vi "Process.vi"(0 "reference in":refnum<class "Graph.lvclass">, 5 "error in":errorcluster) -> (14 "reference out":refnum<class "Graph.lvclass">, 19 "error out":errorcluster)   [LabVIEW 2023, in "Graph.lvclass"]
uses:
  Graph.lvclass
  <vilib>/Utility/SystemLogging/NI_SystemLogging.lvlib
panel:
  out "error info":errorcluster
  out "Last Command":string
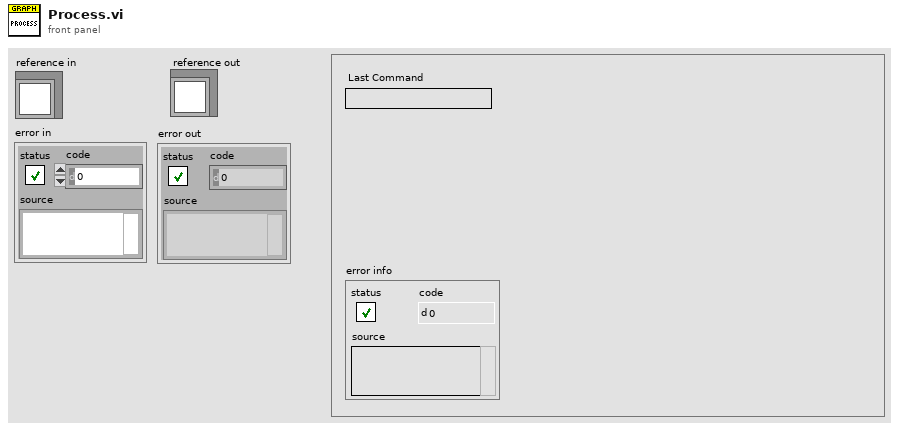
[diagram p1: front panel]
types:
  T1 = cluster{"Core":cluster{"Timeout":i32, "Events":cluster{"EventsToProcess":refnum<event-registration>}, "EventFromProcess":refnum<user-event>, "ProcessSyncQueue":refnum<queue>, "QueueFromProcess":refnum<queue>, "Command":string, "Data":variant}}
  T2 = enum32{"Invalid", "Standard", "Closed", "Hidden", "Minimized", "Maximized"}
  T3 = cluster{"EventsToProcess":refnum<event-registration>}
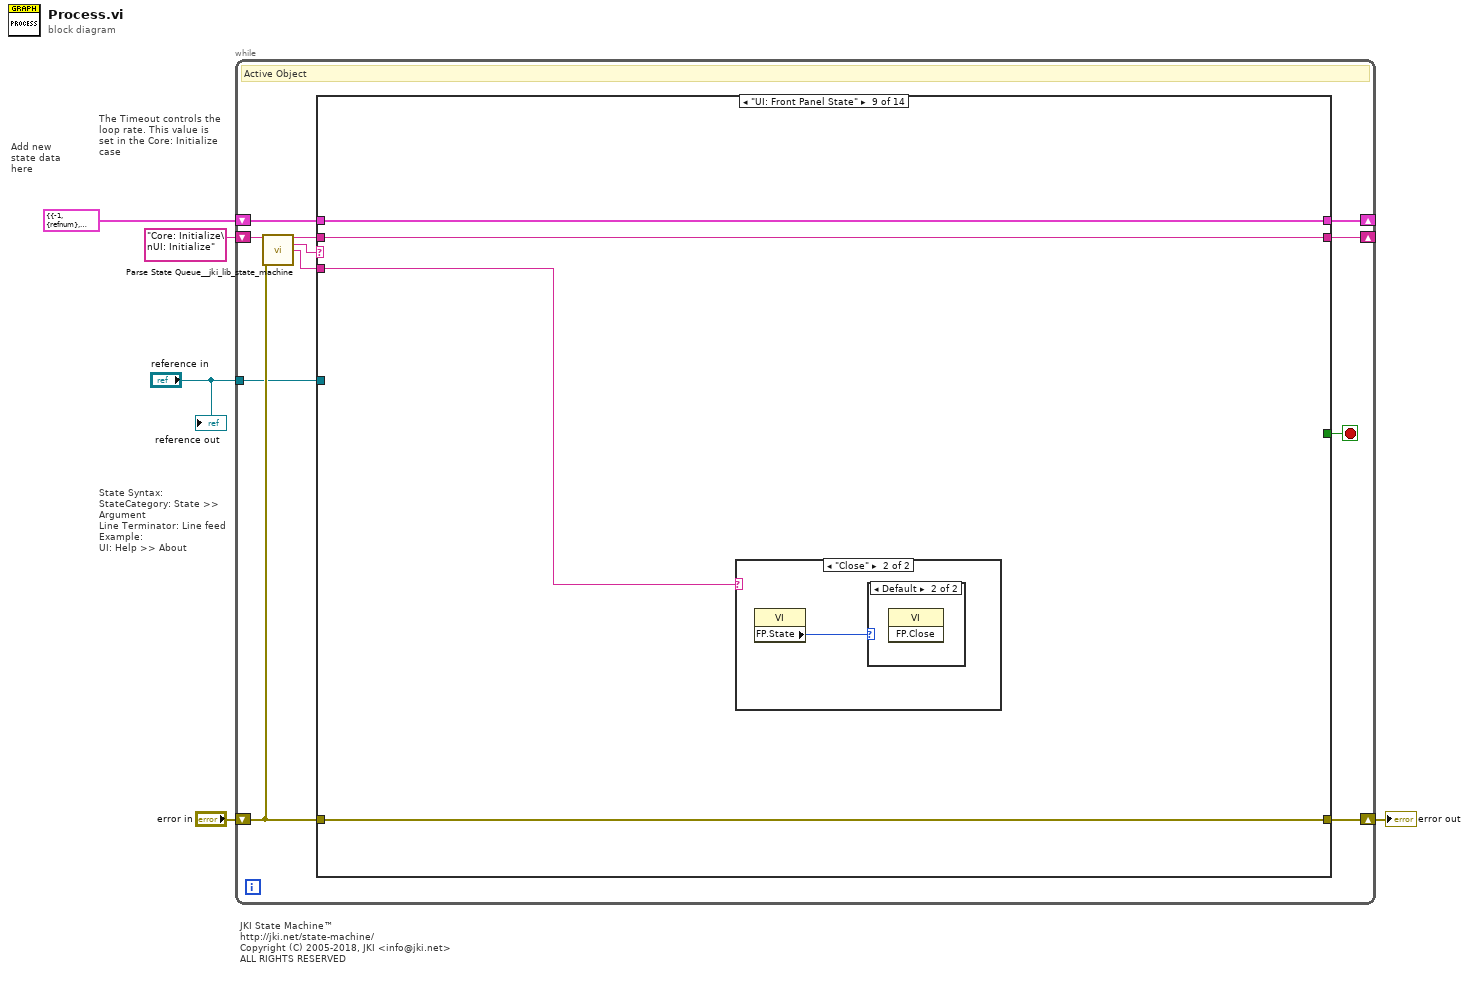
[diagram p0: block diagram]
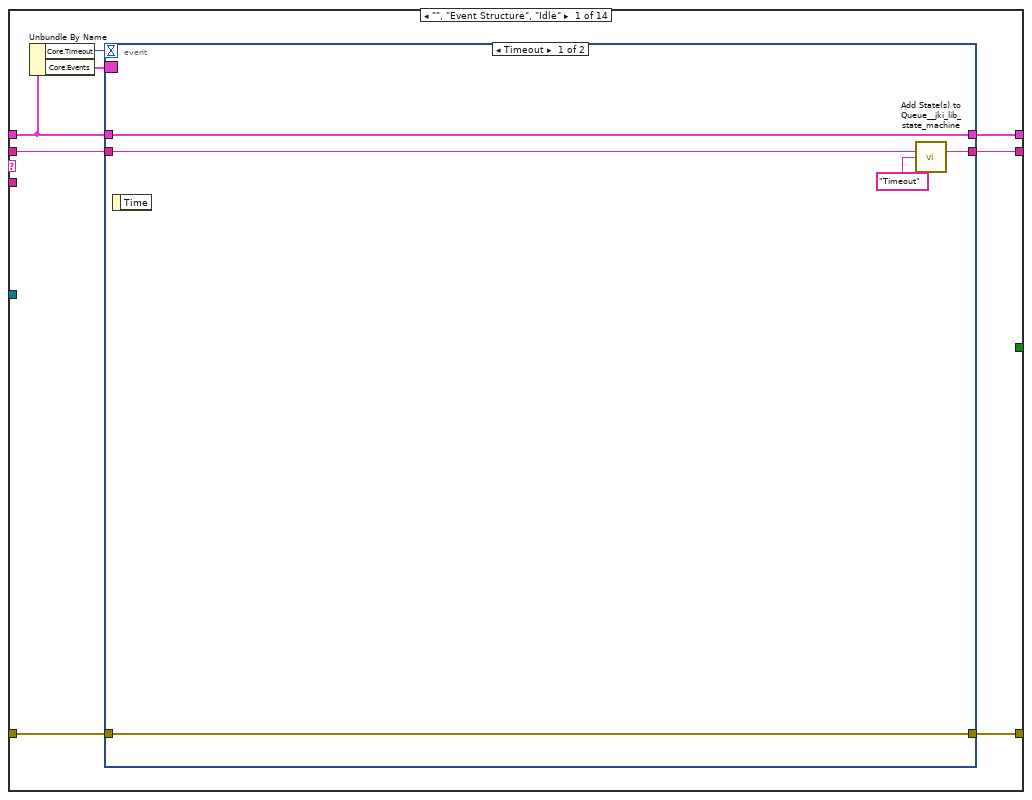
[diagram p2: hidden frame]
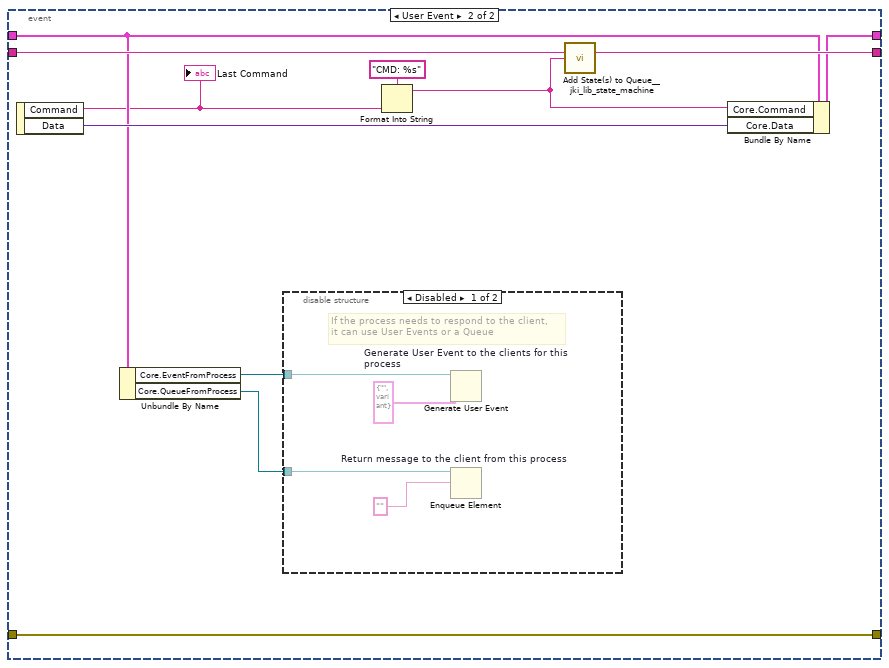
[diagram p3: hidden frame]
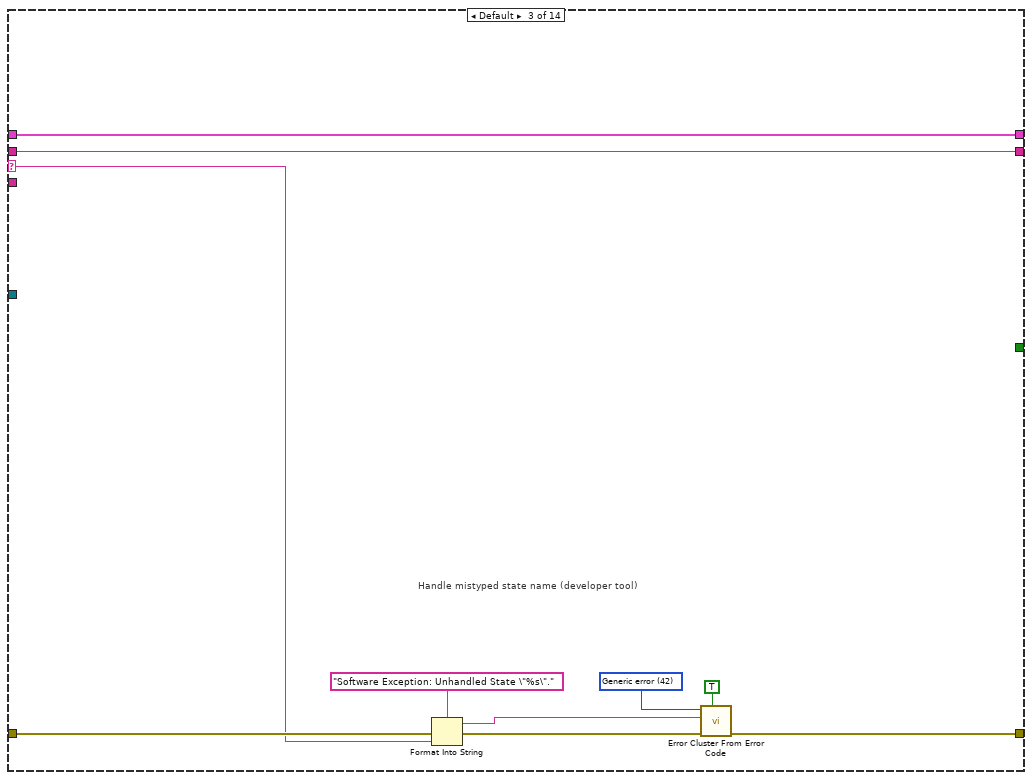
[diagram p6: hidden frame]
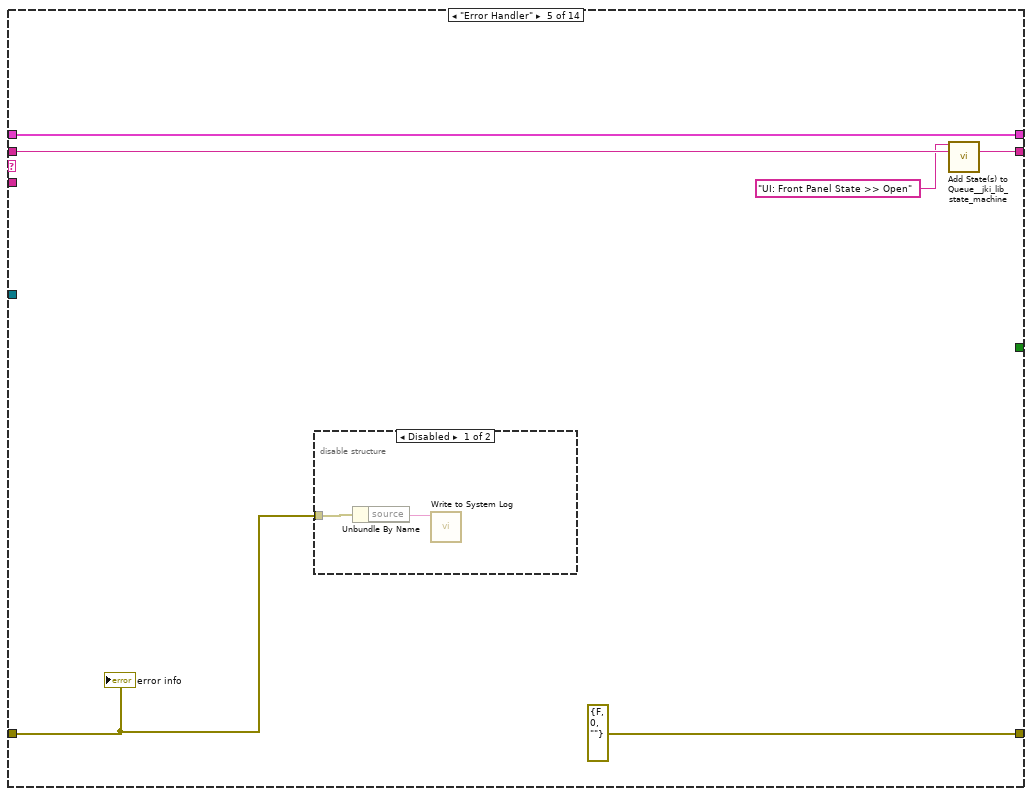
[diagram p8: hidden frame]
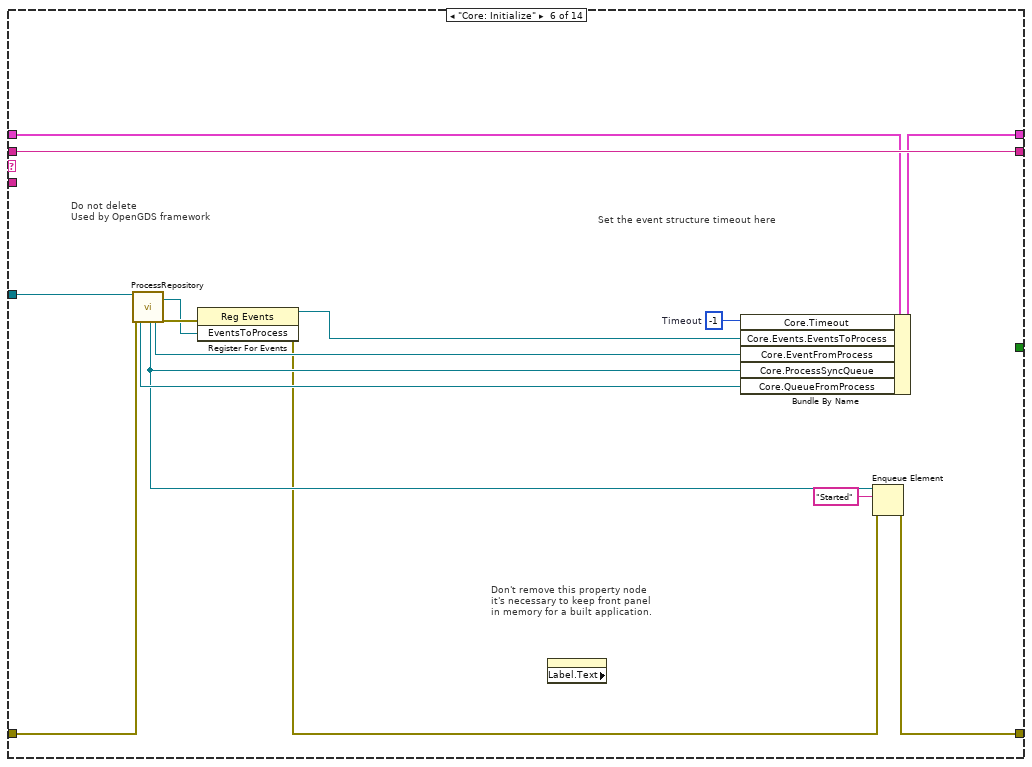
[diagram p10: hidden frame]
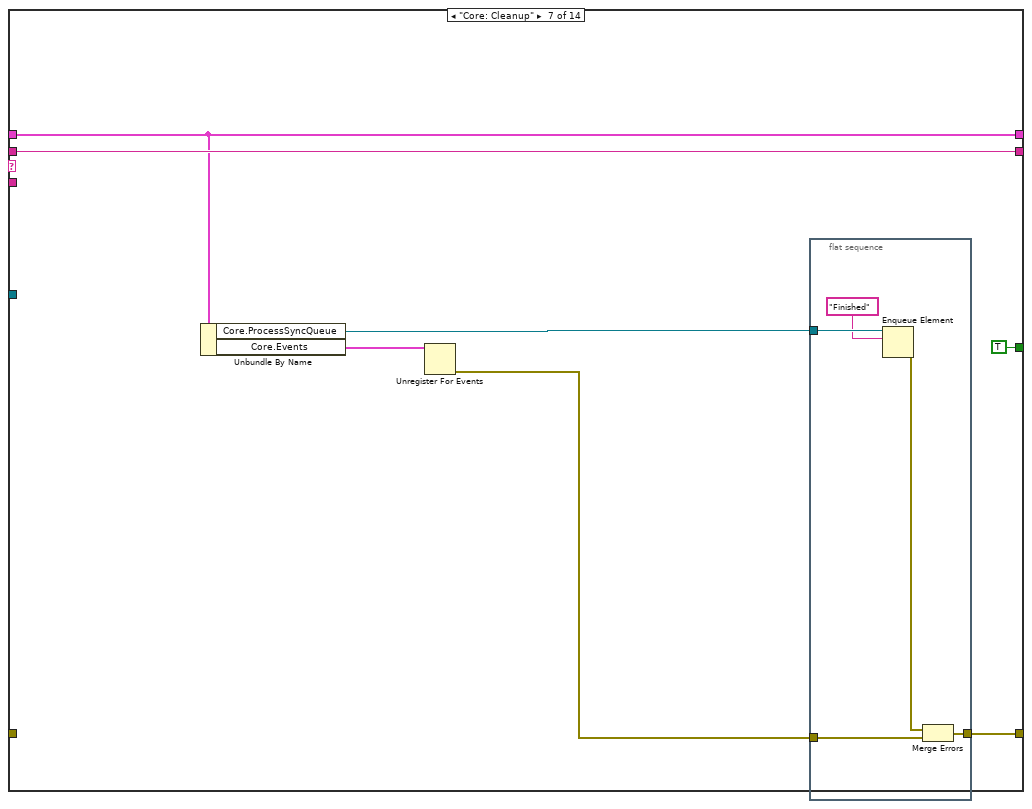
[diagram p11: hidden frame]
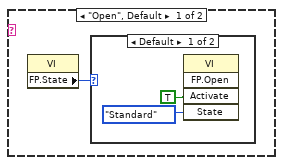
[diagram p13: hidden frame]
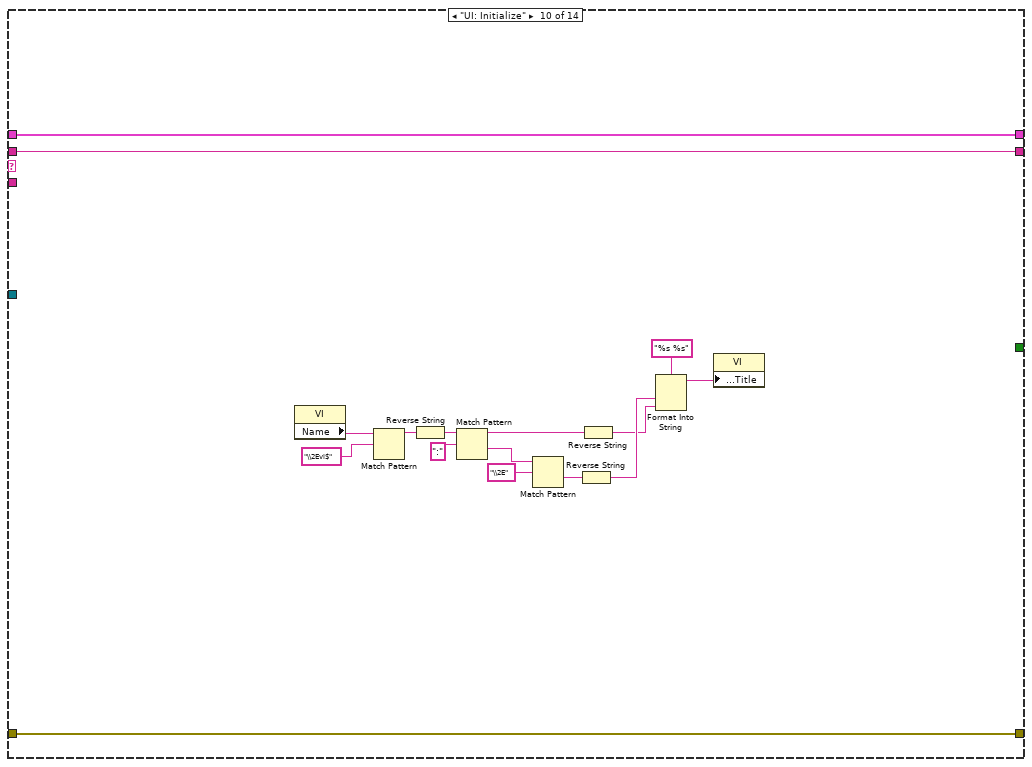
[diagram p16: hidden frame]
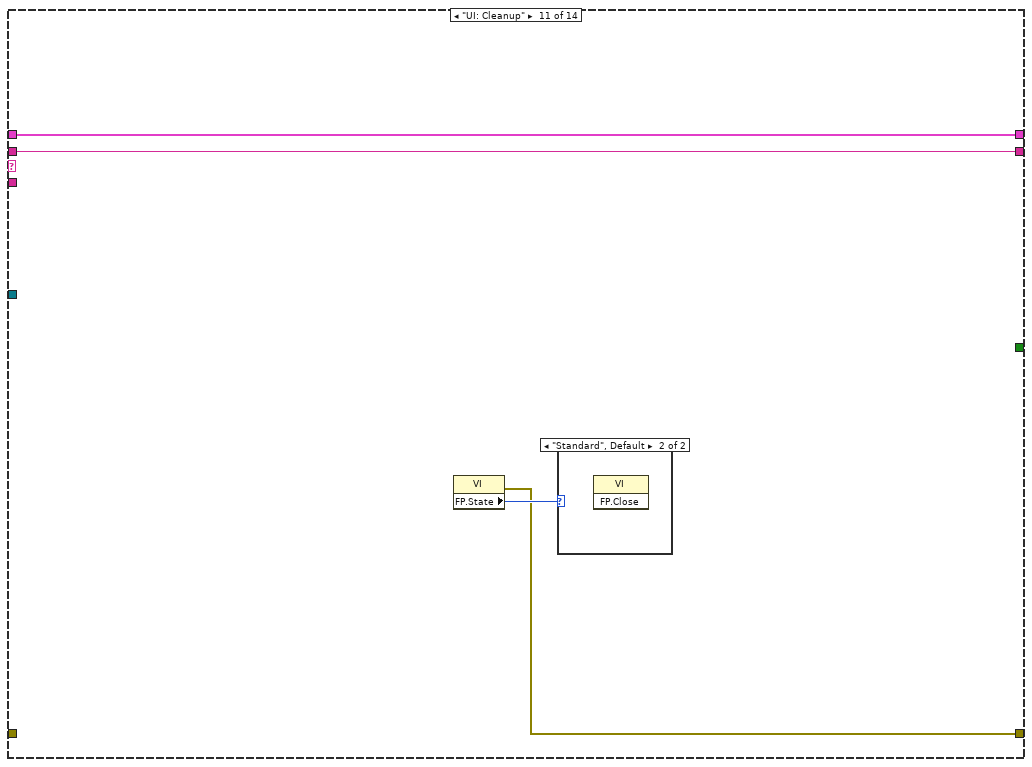
[diagram p17: hidden frame]
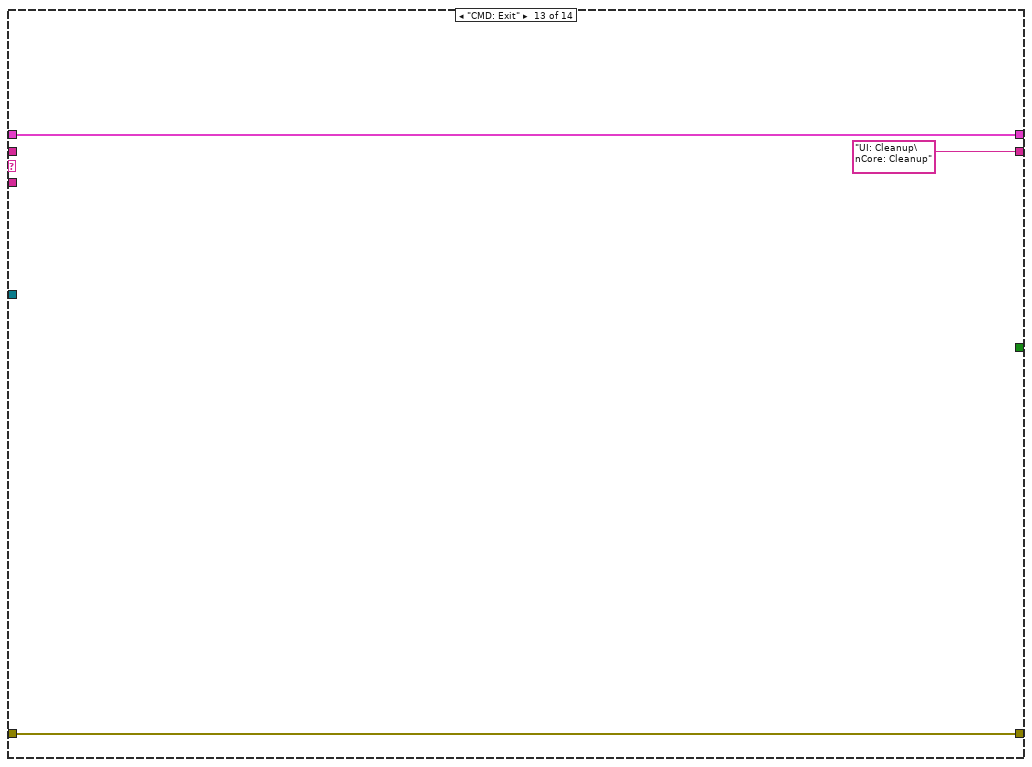
[diagram p20: hidden frame]
diagram:
  # "Add new state data here"
  # "JKI State Machine™\nhttp://jki.net/state-machine/\nCopyright (C) 2005-2018, JKI <info@jki.net>\nALL RIGHTS RESERVED"
  # "State Syntax:\nStateCategory: State >> Argument\nLine Terminator: Line feed\nExample:\nUI: Help >> About"
  # "The Timeout controls the loop rate. This value is set in the Core: Initialize case"
  n1 = while {
    shift-right: [w15] -> w4
    shift-left: "error in" -> [w16]
    shift-right: [w8] -> _
    shift-left: "Core: Initialize\nUI: Initialize" ("States Out") -> [w11]
    shift-right: [w14] -> _
    shift-left: T1 {"Core"={"Timeout"=-1, "Events"={"EventsToProcess"=refnum}, "EventFromProcess"=refnum, "ProcessSyncQueue"=refnum, "QueueFromProcess"=refnum, "Command"="", "Data"=variant}} ("LocalVariables") -> [w13]
    tunnel: "reference in" -> [w6]
    stop <- w7 stop-if-true
    # "Active Object"
    n2 = call <vilib>:"Parse State Queue__jki_lib_state_machine.vi"("State Queue"=w11, "Error In (no error)"=w16) -> ("Remaining States"=w10:string, "Current State"=w12:string, "Arguments"=w9:string)  [unwired: 11 in]
    n3 = case shown="\"UI: Front Panel State\"" w12 {
      selector: w12 -> [_ _ w48 _ _ _ _ _ _ _ _ _ _ _]
      tunnel: w16 -> [w18 w47 w50 w60 w62 w79 _ w98 w99 w122 _ w129 w132 w139]
      tunnel: [w19 w47 w49 w60 errorcluster {"status"=FALSE, "code"=0, "source"=""} ("error constant") w83 w86 w98 w99 w122 w123 w129 w132 w139] -> w15
      tunnel: [w24 w46 w57 w59 w66 w81 w87 w97 w101 w114 w124 w128 w131 w138] -> w14
      tunnel: w13 -> [w20 w46 w57 w59 w66 w80 w87 w97 w101 w114 w124 w128 w131 w138]
      tunnel: w10 -> [w22 w45 w56 w58 w65 w82 w90 w96 w102 w121 w126 w127 _ w137]
      tunnel: w9 -> [_ _ _ _ _ _ _ _ w100 _ _ _ _ w134]
      tunnel: [w21 w45 w56 w58 w64 w82 w90 w96 w102 w121 w126 w127 "UI: Cleanup\nCore: Cleanup" ("State(s) at Back (\"\")") w136] -> w8
      tunnel: [_ _ _ _ _ _ TRUE _ _ _ _ _ _ _] -> w7
      tunnel: w6 -> [_ _ _ _ _ w78 _ _ _ _ _ _ _ _]
      frame "", "Event Structure", "Idle" {
        n4 = Unbundle By Name(w20) -> ("Core.Timeout"=w17:i32, "Core.Events"=w23:T3)
        n5 = event shown="[0] Timeout" {
          selector: w23 -> [_ _]
          dyn-events: _ -> [_ _]
          timeout: w17 -> [_ _]
          tunnel: w20 -> [w29 w33]
          tunnel: [w29 w38] -> w24
          tunnel: [w27 w40] -> w21
          tunnel: w22 -> [w28 w39]
          tunnel: [w25 w34] -> w19
          tunnel: w18 -> [w25 w34]
          event Timeout {
            n6 = event-data() -> ()  [unwired: 1 in, 1 out]
            n7 = call <vilib>:"Add State(s) to Queue__jki_lib_state_machine.vi"("State(s) in (\"\")"=w28, "State(s) at Back (\"\")"="Timeout" ("State(s) at Back (\"\")")) -> ("States Out"=w27:string)  [unwired: 13 in]
          }
          event User Event {
            n8 = event-data() -> ("Command"=w31:string, "Data"=w37:variant)  [unwired: 1 in]
            "Last Command" <- w31
            n9 = Unbundle By Name(w33) -> ("Core.EventFromProcess"=w36:refnum<user-event>, "Core.QueueFromProcess"=w35:refnum<queue>)
            n10 = disable-structure shown="Disabled" {
              disable-tunnel: w36 -> [w44 _]
              disable-tunnel: w35 -> [w43 _]
              frame Disabled {
                # "If the process needs to respond to the client,\nit can use User Events or a Queue"
                n11 = Generate User Event "Generate User Event to the clients for this process"(user event=w44, event data cluster=cluster{"Command":string, "Data":variant} {"Command"="", "Data"=variant} ("event data")) -> ()  [unwired: 2 in, 2 out]
                n12 = Enqueue Element "Return message to the client from this process"(queue=w43, element="") -> ()  [unwired: 2 in, 3 out]
              }
              frame Enabled {
              }
            }
            n13 = Format Into String(format string="CMD: %s", w31) -> (resulting string=w30:string)  [unwired: 2 in, 1 out]
            n14 = call <vilib>:"Add State(s) to Queue__jki_lib_state_machine.vi"("State(s) in (\"\")"=w39, "State(s) at Back (\"\")"=w30) -> ("States Out"=w40:string)  [unwired: 13 in]
            n15 = Bundle By Name(cluster=w33, "Core.Command"=w30, "Core.Data"=w37) -> (w38:T1)
          }
        }
      }
      frame "---------- Core ----------" {
      }
      frame Default {
        w54 = 42 items=["No error", "Argument error", "Memory is full", "Out of zone", "End of file", "File already open", "Generic file I/O error", "File not found", "File permission error", "Disk is full", "Duplicate path", "Too many files open", "System feature not enabled", "Resource file not found", "Cannot add resource", "Resource not found", "Image not found", "Image memory error", "Pen does not exist", "Config type invalid", "Config token not found", "Config parse error", "Config memory error", "Bad external code format", "Bad external code offset", "External code not present", "Null window", "Destroy window error", "Null menu", "Print aborted", "Bad print record", "Print driver error", "Windows error during printing", "Memory error during printing", "Print dialog error", "Generic print error", "Invalid device refnum", "Device not found", "Device parameter error", "Device unit error", "Cannot open device", "Device call aborted", "Generic error", "Cancelled by user", "Object ID too low", "Object ID too high", "Object not in heap", "Unknown heap", "Unknown object (invalid DefProc)", "Unknown object (DefProc not in table)", "Message out of range", "Invalid (null) method", "Unknown message", "Manager call not supported", "Bad address", "Network operation in progress", "Network operation timed out", "Connection is busy", "Network attribute not supported", "Network error", "Address in use", "System out of memory", "Connection aborted", "Connection refused", "Not connected", "Already connected", "Connection closed", "Initialization error (interapplication manager)", "Bad occurrence", "Wait on unbound occurrence handler", "Occurrence queue overflow", "Datalog type conflict", "Unused", "Unrecognized type (interapplication manager)", "Memory corrupt", "Failed to make temporary DLL", "Old CIN version", "Drag socket not found", "Failed to load drop-object", "Failed to register OLE object", "Failed to release OLE object", "Format specifier type mismatch", "Unknown format specifier", "Too few format specifiers", "Too many format specifiers", "Scan failed", "Newer CIN version", "Error converting to variant", "Runtime menu error", "Password tampered", "Variant attribute not found", "Incompatible variant data type", "Event data is not available", "Event Store is not present", "Occurrence is not found", "Event Queue is not created", "Event info is not available", "Refnum passed is NULL", "Error retrieving Class GUID", "Error retrieving CoClass GUID", "Error retrieving TypeLib GUID.", "Bad built application magic bytes.", "Specific driver is different from the specific driver associated with the Logical Name.", "There is no session opened to the class driver.", "Max Error", "MAX - Error with config objects", "MAX - Error loading configuration", "MAX - Group not supported"]
        # "Handle mistyped state name (developer tool)"
        n16 = Format Into String(format string="Software Exception: Unhandled State \"%s\"." ("message"), error in=w50, w48) -> (resulting string=w53:string, error out=w52:errorcluster)  [unwired: 1 in]
        n17 = call <vilib>:"Error Cluster From Error Code.vi"("show call chain? (False)"=TRUE, "error in (no error)"=w52, "error message (\"\")"=w53, "error code (0)"=w54) -> ("error out"=w49:errorcluster)  [unwired: 5 in]
      }
      frame "Timeout" {
      }
      frame "Error Handler" {
        n18 = disable-structure shown="Disabled" {
          disable-tunnel: w62 -> [w68 _]
          frame Disabled {
            n19 = Unbundle By Name(w68) -> ("source"=w67:string)
            n20 = call <vilib>:"Write to System Log.vi"("message"=w67) -> ()  [unwired: 10 in, 1 out]
          }
          frame Enabled {
          }
        }
        n21 = call <vilib>:"Add State(s) to Queue__jki_lib_state_machine.vi"("State(s) in Front (\"\")"="UI: Front Panel State >> Open" ("State(s) at Back (\"\")"), "State(s) in (\"\")"=w65) -> ("States Out"=w64:string)  [unwired: 13 in]
        "error info" <- w62
      }
      frame "Core: Initialize" {
        w69 = -1  # Timeout
        # "Do not delete\nUsed by OpenGDS framework"
        # "Set the event structure timeout here"
        # "Don't remove this property node\nit's necessary to keep front panel\nin memory for a built application."
        # "Template created by VI Technologies"
        n22 = call "ProcessRepository.vi"("reference in"=w78, "Error In"=w79) -> ("QueueFromProcess"=w73:refnum<queue>, "ProcessSyncQueue"=w71:refnum<queue>, "EventFromProcess"=w74:refnum<user-event>, "EventsToProcess"=w76:refnum<user-event>, "Error Out"=w77:errorcluster)  [unwired: 10 in, 3 out]
        n23 = register-events(error in=w77, w76) -> (reference out=w75:refnum<event-registration>, error out=w70:errorcluster)  [unwired: 1 in]
        n24 = property on="reference in" class="LVClassControl (strict)" props=["Label", "Text"]() -> ()  [unwired: 2 in, 3 out]
        n25 = Bundle By Name(cluster=w80, "Core.Timeout"=w69, "Core.Events.EventsToProcess"=w75, "Core.EventFromProcess"=w74, "Core.ProcessSyncQueue"=w71, "Core.QueueFromProcess"=w73) -> (w81:T1)
        n26 = Enqueue Element(queue=w71, element="Started", error in (no error)=w70) -> (error out=w83:errorcluster)  [unwired: 1 in, 2 out]
      }
      frame "Core: Cleanup" {
        n27 = Unbundle By Name(w87) -> ("Core.ProcessSyncQueue"=w88:refnum<queue>, "Core.Events"=w85:T3)
        n28 = Unregister For Events(event registration refnum=w85) -> (error out=w84:errorcluster)  [unwired: 1 in]
        n29 = flat-sequence {
          tunnel: [w94] -> w86
          tunnel: w88 -> [w93]
          tunnel: w84 -> [w92]
          frame #0 {
            n30 = Enqueue Element(queue=w93, element="Finished") -> (error out=w95:errorcluster)  [unwired: 2 in, 2 out]
            n31 = Merge Errors(w95, w92) -> (w94:errorcluster)
          }
        }
      }
      frame "---------- UI ----------" {
      }
      frame "UI: Front Panel State" {
        n32 = case shown="\"Close\"" w100 {
          frame "Open", Default {
            n33 = property class="VI"() -> ("FP.State"=w103:T2)  [unwired: 2 in, 2 out]
            n34 = case shown="Default" w103 {
              frame Default {
                n35 = invoke class="VI" method="FP.Open"("Activate"=TRUE, "State"=T2."Standard") -> ()  [unwired: 3 in, 5 out]
              }
              frame "Standard" {
              }
            }
          }
          frame "Close" {
            n36 = property class="VI"() -> ("FP.State"=w106:T2)  [unwired: 2 in, 2 out]
            n37 = case shown="Default" w106 {
              frame "Closed" {
              }
              frame Default {
                n38 = invoke class="VI" method="FP.Close"() -> ()  [unwired: 3 in, 3 out]
              }
            }
          }
        }
      }
      frame "UI: Initialize" {
        n39 = property class="VI"() -> ("Name"=w120:string)  [unwired: 2 in, 2 out]
        n40 = Match Pattern(string=w120, regular expression="\\2Evi$") -> (before substring=w118:string)  [unwired: 1 in, 3 out]
        n41 = Reverse String(1:w118) -> (0:w117:string)
        n42 = Match Pattern(string=w117, regular expression=":") -> (before substring=w115:string, after substring=w113:string)  [unwired: 1 in, 2 out]
        n43 = Match Pattern(string=w113, regular expression="\\2E") -> (after substring=w111:string)  [unwired: 1 in, 3 out]
        n44 = Reverse String(1:w111) -> (0:w110:string)
        n45 = Reverse String(1:w115) -> (0:w109:string)
        n46 = Format Into String(format string="%s %s", w110, w109) -> (resulting string=w108:string)  [unwired: 2 in, 1 out]
        n47 = property class="VI"("Front Panel.Title"=w108) -> ()  [unwired: 2 in, 2 out]
      }
      frame "UI: Cleanup" {
        n48 = property class="VI"() -> (error out=w123:errorcluster, "FP.State"=w125:T2)  [unwired: 2 in, 1 out]
        n49 = case shown="\"Standard\", Default" w125 {
          frame "Closed" {
          }
          frame "Standard", Default {
            n50 = invoke class="VI" method="FP.Close"() -> ()  [unwired: 3 in, 3 out]
          }
        }
      }
      frame "---------- CMD ----------" {
      }
      frame "CMD: Exit" {
      }
      frame "CMD: Front Panel State" {
        n51 = Format Into String(format string="UI: Front Panel State>>%s" ("string"), w134) -> (resulting string=w133:string)  [unwired: 2 in, 1 out]
        n52 = call <vilib>:"Add State(s) to Queue__jki_lib_state_machine.vi"("State(s) in (\"\")"=w137, "State(s) at Back (\"\")"=w133) -> ("States Out"=w136:string)  [unwired: 13 in]
      }
    }
  }
  "error out" <- w4
  "reference out" <- "reference in"
